vi "GF_ArmAgilent.vi"(0 "Agilent Control In":T1={"Trig?"=FALSE, "VISA session"="Agilent6034", "Setup to Load"="2", "Timeout (ms)"=40000, "Desired Samp"=enum."1000", "Captured Samp"=11, "Desired Channels"=[{"Chan Index"=enum."Channel1", "Name"="Chan1Test", "Samples"=0}, {"Chan Index"=enum."Channel2", "Name"="Chan2Test", "Samples"=0}, {"Chan Index"=enum."Channel3", "Name"="Chan3Test", "Samples"=0}, {"Chan Index"=enum."Channel4", "Name"="Chan4Test", "Samples"=0}]}) -> (1 "Agilent Control Out":T1={"Trig?"=FALSE, "VISA session"="Agilent6034", "Setup to Load"="2", "Timeout (ms)"=40000, "Desired Samp"=enum."1000", "Captured Samp"=11, "Desired Channels"=[{"Chan Index"=enum."Channel1", "Name"="Chan1Test", "Samples"=0}, {"Chan Index"=enum."Channel2", "Name"="Chan2Test", "Samples"=0}, {"Chan Index"=enum."Channel3", "Name"="Chan3Test", "Samples"=0}, {"Chan Index"=enum."Channel4", "Name"="Chan4Test", "Samples"=0}]}, 2 "Agilent Present":bool=TRUE, 3 "Agilent Setup Error":errorcluster)   [LabVIEW 2009]
uses:
  AgilentControl.ctl
  Channel Config.ctl
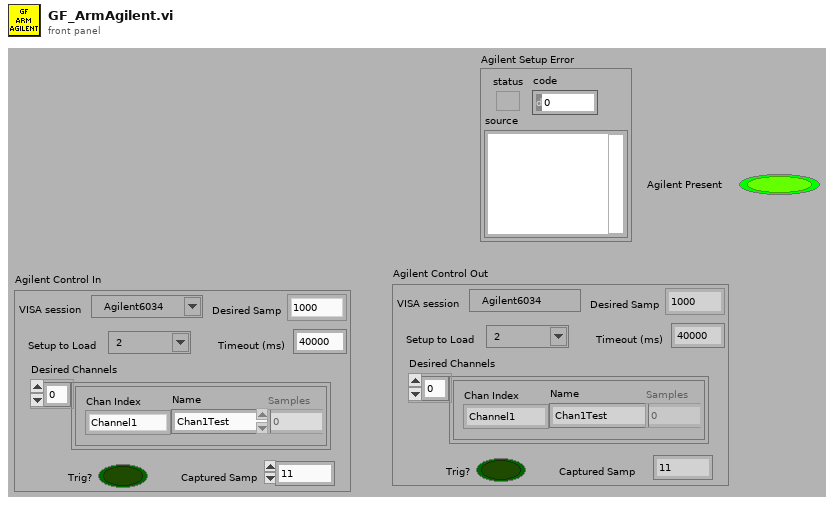
[diagram p1: front panel]
types:
  T1 = typedef "AgilentControl.ctl" = cluster{"Trig?":bool, "VISA session":refnum<visa-resource-name>, "Setup to Load":string, "Timeout (ms)":u32, "Desired Samp":enum32{"100", "250", "500", "1000", "2000", "5000", "10000", "20000", "50000", "100000", "200000", "500000", "1000000", "2000000", "4000000", "8000000"}, "Captured Samp":i32, "Desired Channels":T2[]}
  T2 = typedef "Channel Config.ctl" = cluster{"Chan Index":enum16{"Channel1", "Channel2", "Channel3", "Channel4", "MATH"}, "Name":string, "Samples":i32}
  T3 = enum32{"100", "250", "500", "1000", "2000", "5000", "10000", "20000", "50000", "100000", "200000", "500000", "1000000", "2000000", "4000000", "8000000"}
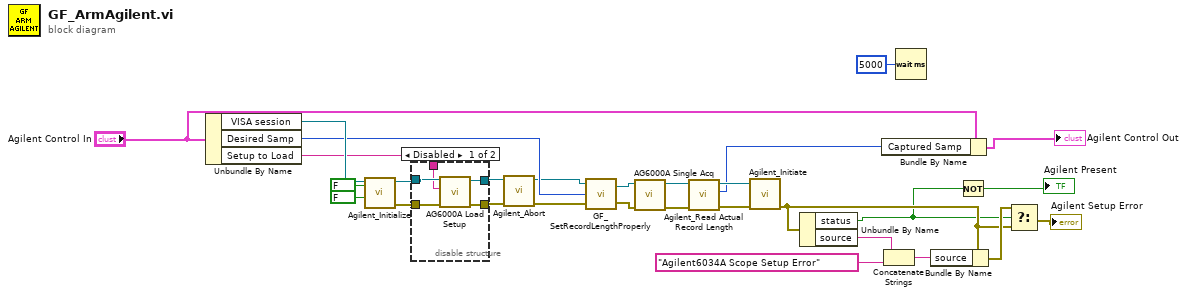
[diagram p0: block diagram]
diagram:
  n1 = Unbundle By Name("Agilent Control In") -> ("VISA session"=w20:refnum<visa-resource-name>, "Desired Samp"=w19:T3, "Setup to Load"=w18:string)
  n2 = call "Agilent_Initialize.vi"("Reset? (T: Yes)"=FALSE, "ID Query? (T: Yes)"=FALSE, "VISA resource name"=w20) -> ("error out"=w28:errorcluster, "VISA resource name out"=w29:refnum<visa-resource-name>)  [unwired: 7 in]
  n3 = disable-structure shown="Disabled" {
    disable-tunnel: [w34 w35] -> w5
    disable-tunnel: [w33 w36] -> w8
    disable-tunnel: w29 -> [w32 w35]
    disable-tunnel: w28 -> [w31 w36]
    disable-tunnel: w18 -> [w30 _]
    frame #0 {
      n4 = call "AG6000A Load Setup.vi"("error in (no error)"=w31, "Setup to Load"=w30, "VISA session"=w32) -> ("error out"=w33:errorcluster, "dup VISA session"=w34:refnum<visa-resource-name>)  [unwired: 7 in]
    }
    frame #1 {
    }
  }
  n5 = call "Agilent_Abort.vi"("error in (no error)"=w8, "VISA resource name"=w5) -> ("error out"=w7:errorcluster, "VISA resource name out"=w6:refnum<visa-resource-name>)  [unwired: 8 in]
  n6 = call "GF_SetRecordLengthProperly.vi"("error in (no error)"=w7, "Num Samples"=w19, "VISA resource name"=w6) -> ("error out"=w22:errorcluster, "VISA resource name out"=w23:refnum<visa-resource-name>)
  n7 = call "AG6000A Single Acq.vi"("error in (no error)"=w22, "VISA session"=w23) -> ("error out"=w24:errorcluster, "dup VISA session"=w25:refnum<visa-resource-name>)  [unwired: 8 in]
  n8 = call "Agilent_Read Actual Record Length.vi"("error in (no error)"=w24, "VISA resource name"=w25) -> ("error out"=w26:errorcluster, "Actual Record Length"=w17:i32, "VISA resource name out"=w27:refnum<visa-resource-name>)  [unwired: 7 in]
  n9 = call "Agilent_Initiate.vi"("error in (no error)"=w26, "VISA resource name"=w27) -> ("error out"=w12:errorcluster)  [unwired: 8 in, 1 out]
  n10 = Unbundle By Name(w12) -> ("status"=w11:bool, "source"=w16:string)
  n11 = Bundle By Name(cluster="Agilent Control In", "Captured Samp"=w17) -> (→"Agilent Control Out":T1)
  n12 = Concatenate Strings(w16, "Agilent6034A Scope Setup Error") -> (w15:string)
  n13 = Wait (ms)(milliseconds to wait=u32 5000) -> ()  [unwired: 1 out]
  n14 = Bundle By Name(cluster=w12, "source"=w15) -> (w13:errorcluster)
  n15 = Not(x=w11) -> (.not. x?=→"Agilent Present":bool)
  n16 = Select(t=w13, s=w11, f=w12) -> (s? t:f=→"Agilent Setup Error":errorcluster)
